vi "json Parse I64 Array - string path.vi"(6 "use default?":bool=TRUE, 8 "error in (no error)":errorcluster, 9 "default":i64[](array[numeric]), 10 "path":string, 11 "JSON Document in":refnum<class "JSON Document.lvclass">) -> (0 "error out":errorcluster, 1 "defaulted?":bool, 2 "value":i64[](array[numeric]), 3 "JSON Document out":refnum<class "JSON Document.lvclass">, 4 "elements defaulted?":bool[](array[boolean]))   [LabVIEW 2015, in "JSON Document.lvclass"]
uses:
  JSON Document.lvclass
  json Parse I64 - string path.vi
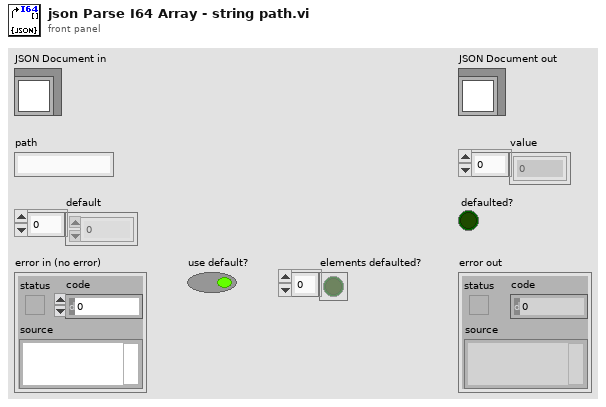
[diagram p1: front panel]
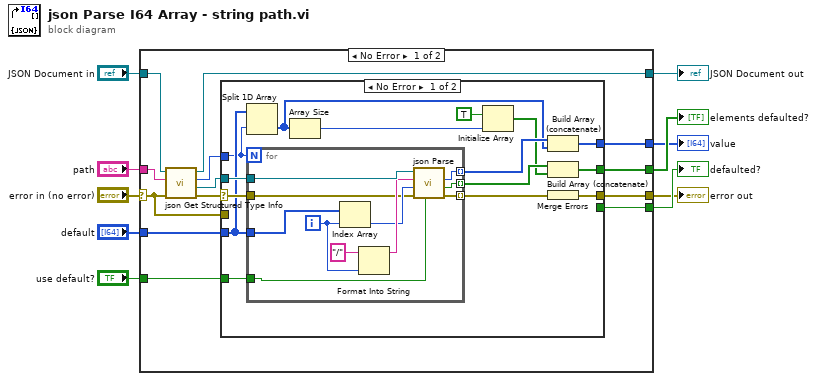
[diagram p0: block diagram]
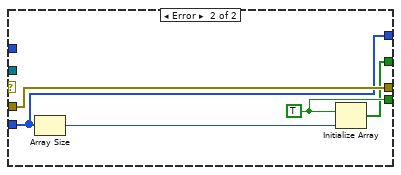
[diagram p2: hidden frame]
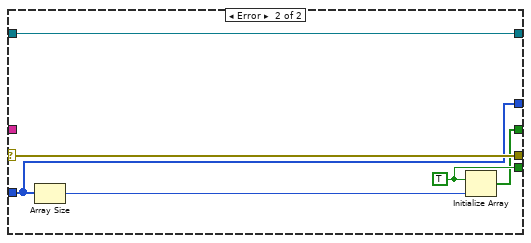
[diagram p3: hidden frame]
diagram:
  n1 = case shown="No Error" "error in (no error)" {
    selector: "error in (no error)" -> [w23 w60]
    tunnel: [w22 w60] -> w2
    tunnel: [w14 w59] -> w6
    tunnel: "JSON Document in" -> [w15 w59]
    tunnel: "default" -> [w20 w58]
    tunnel: "path" -> [w13 _]
    tunnel: [w21 w58] -> w3
    tunnel: [w19 w56] -> w5
    tunnel: [w12 w55] -> w4
    tunnel: "use default?" -> [w11 _]
    frame No Error {
      n2 = call "json Get Structured Type Info.vi"("error in (no error)"=w23, "path"=w13, "JSON Document in"=w15) -> ("error out"=w17:errorcluster, "value out"=w16:refnum<class "JSON Document.lvclass">, "count"=w18:i32, "JSON Document out"=w14:refnum<class "JSON Document.lvclass">)  [unwired: 5 in]
      n3 = case shown="No Error" w17 {
        selector: w17 -> [w38 _]
        tunnel: [w32 w53] -> w21
        tunnel: w18 -> [w25 _]
        tunnel: w20 -> [w34 w53]
        tunnel: [w36 w54] -> w22
        tunnel: w23 -> [_ w54]
        tunnel: w16 -> [w35 _]
        tunnel: [_ w51] -> w19
        tunnel: [w26 w50] -> w12
        tunnel: w11 -> [w24 _]
        frame No Error {
          n4 = Split 1D Array(array=w34, index=w25) -> (second subarray=w31:i64[])  [unwired: 1 out]
          n5 = for {
            N: w25 -> [_]
            tunnel: [w43] -> w37 mode=indexing
            tunnel: [w42] -> w33 mode=indexing
            tunnel: w34 -> [w48]
            tunnel: w38 -> [w44]
            tunnel: w35 -> [w47]
            tunnel: [w40] -> w28 mode=indexing
            tunnel: w24 -> [w39]
            i -> [w41]
            n6 = Index Array(array=w48, index=w41) -> (element=w45:i64)
            n7 = Format Into String(initial string="/", w41) -> (resulting string=w46:string)  [unwired: 2 in, 1 out]
            n8 = call-poly "json Parse.vi"("use default?"=w39, "error in (no error)"=w44, "default"=w45, "path"=w46, "JSON Document in"=w47) -> ("error out"=w43:errorcluster, "defaulted?"=w40:bool, "value"=w42:i64)  [unwired: 3 in, 1 out]
          }
          n9 = Array Size(array=w31) -> (size(s)=w30:i32)
          n10 = Initialize Array(TRUE ("found?"), w30) -> (w27:bool[])
          n11 = Build Array (concatenate)(w33, w31) -> (w32:i64[])
          n12 = Build Array (concatenate)(w28, w27) -> (w26:bool[])
          n13 = Merge Errors(w37) -> (w36:errorcluster)
        }
        frame Error {
          w51 = TRUE ("found?")
          n14 = Array Size(array=w53) -> (size(s)=w52:i32)
          n15 = Initialize Array(w51, w52) -> (w50:bool[])
        }
      }
    }
    frame Error {
      w56 = TRUE ("found?")
      n16 = Array Size(array=w58) -> (size(s)=w57:i32)
      n17 = Initialize Array(w56, w57) -> (w55:bool[])
    }
  }
  "error out" <- w2
  "JSON Document out" <- w6
  "value" <- w3
  "defaulted?" <- w5
  "elements defaulted?" <- w4
